vi "ID check.vi"() -> ()   [LabVIEW 2015]
panel:
  out "hi(x)":u16
  in  "Numeric Control":u32=1280507904
  out "unsigned byte array":u8[](array[numeric]) format="%.0f (x%x) (%s)"
  out "(hi.lo)":u16 format="%.0d (x%x)"
  in  "String":string="LS"
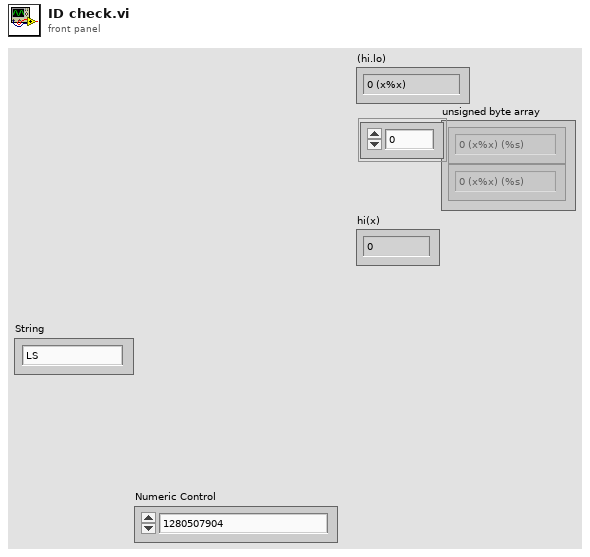
[diagram p1: front panel]
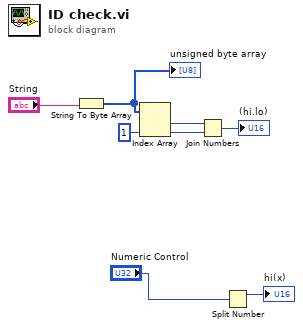
[diagram p0: block diagram]
diagram:
  n1 = String To Byte Array(string="String") -> (unsigned byte array=w7:u8[])
  "unsigned byte array" <- w7
  n2 = Index Array(array=w7, index #2=1 ("index")) -> (element #1=w5:u8, element #2=w4:u8)  [unwired: 1 in]
  n3 = Join Numbers(hi=w5, lo=w4) -> ((hi.lo)=→"(hi.lo)":u16)
  n4 = Split Number(x="Numeric Control") -> (hi(x)=→"hi(x)":u16)  [unwired: 1 out]
